vi "Check CSM Modules Exist Or Not.vi"(8 "error in":errorcluster, 11 "CSM names in":string[](array[string])) -> (0 "error out":errorcluster, 2 "Debug string":string, 3 "All Modules Exist?":bool)   [LabVIEW 2017, in "CSM-Testcase.lvlib"]
uses:
  CSM-Testcase.lvlib
  src/user.lib/_NEVSTOP/Communicable State Machine(CSM)/Communicable State Machine.lvlib
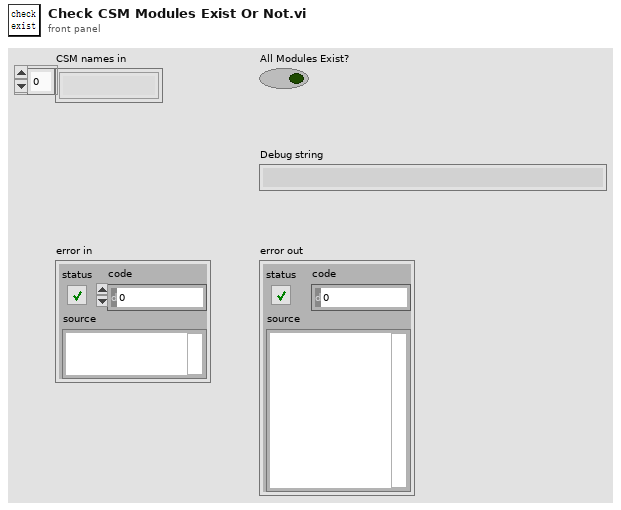
[diagram p1: front panel]
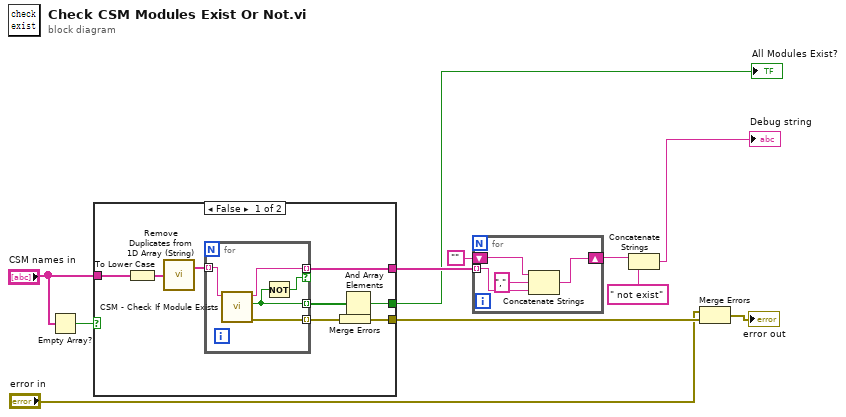
[diagram p0: block diagram]
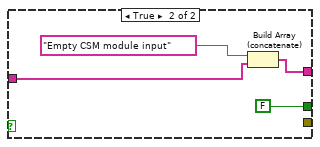
[diagram p2: hidden frame]
diagram:
  n1 = Empty Array?(array="CSM names in") -> (empty?=w2:bool)
  n2 = case shown="False" w2 {
    tunnel: "CSM names in" -> [w18 w26]
    tunnel: [w16 w25] -> w7
    tunnel: [w15 _] -> w6
    tunnel: [w13 FALSE] -> w5
    frame False {
      n3 = To Lower Case(string=w18) -> (all lower case string=w19:string[])
      n4 = call "Remove Duplicates from 1D Array (String).vi"("Input Array"=w19) -> ("Output Array"=w17:string[])  [unwired: 1 out]
      n5 = for {
        tunnel: [w22] -> w12 mode=indexing
        tunnel: [w24] -> w14 mode=indexing
        tunnel: [w23] -> w16 mode=indexing if=w21
        tunnel: w17 -> [w20] mode=indexing
        n6 = call "CSM - Check If Module Exists.vi"("CSM Name"=w20) -> ("error out"=w24:errorcluster, "Exist?"=w22:bool, "CSM Name (Dup)"=w23:string)  [unwired: 8 in]
        n7 = Not(x=w22) -> (.not. x?=w21:bool)
      }
      n8 = Merge Errors(w14) -> (w15:errorcluster)
      n9 = And Array Elements(Boolean array=w12) -> (logical AND=w13:bool)
    }
    frame True {
      n10 = Build Array (concatenate)("Empty CSM module input", w26) -> (w25:string[])
    }
  }
  "All Modules Exist?" <- w5
  n11 = for {
    tunnel: w7 -> [w32] mode=indexing
    shift-right: [w29] -> w9
    shift-left: "" -> [w30]
    n12 = Concatenate Strings(w30, ",", w32) -> (w29:string)
  }
  n13 = Concatenate Strings(w9, " not exist" ("string")) -> (→"Debug string":string)
  n14 = Merge Errors("error in", w6) -> (→"error out":errorcluster)
